vi "Do Action.vi"(7 "Assert Service Enqueuer":refnum<class "Message Enqueuer.lvclass">, 8 "error in (no error)":errorcluster, 11 "UDP Listener in":refnum<class "UDP Listener.lvclass">) -> (0 "error out":errorcluster, 3 "UDP Listener out":refnum<class "UDP Listener.lvclass">)   [LabVIEW 2016, in "Assert API Components.lvlib" / "Assert Service.lvlib" / "UDP Listener.lvclass"]
uses:
  UDP Listener.lvclass
  C:/Users/ukhornp/Documents/Projects/actor_assert_api/Core/Assert Service/Service Actions/Service Action Base.lvclass
  <vilib>/ActorFramework/Message Enqueuer/Message Enqueuer.lvclass
  UDP Listener.lvclass/UDP Listener.ctl
  <vilib>/NI/STM/SubVIs/MetaDataElement.ctl
  Assert Service Messages/New P2P UDP Link Msg/New P2P UDP Link Msg.lvclass/New P2P UDP Link Msg.ctl
  <vilib>/ActorFramework/Message Enqueuer/Message Enqueuer.lvclass/Message Enqueuer.ctl
  <vilib>/NI/STM/UDP/Write Meta Data (UDP Ref).vi
  <vilib>/NI/STM/UDP/Get Connection Reference (UDP).vi
  <vilib>/ActorFramework/Message Enqueuer/Enqueue.vi
  Assert Service Messages/New P2P UDP Link Msg/New P2P UDP Link Msg.lvclass
  C:/Program Files (x86)/National Instruments/LabVIEW 2016/vi.lib/ActorFramework/Message/Message.lvclass
  <vilib>/NI/STM/UDP/Write Meta Data (UDP Clst).vi
  <vilib>/NI/STM/UDP/Read Message (UDP).vi
  <vilib>/NI/STM/UDP/Write Message (UDP).vi
  <vilib>/Utility/LVClass/Get LV Class Name.vi
  <resource>/AFDebug/Generate Trace for Message.vi
  <vilib>/ActorFramework/Message Priority Queue/Priority Enqueue.vi
  <vilib>/NI/STM/NI STM.lvlib
  Service Action Base.lvclass
panel:
  out "data string":string
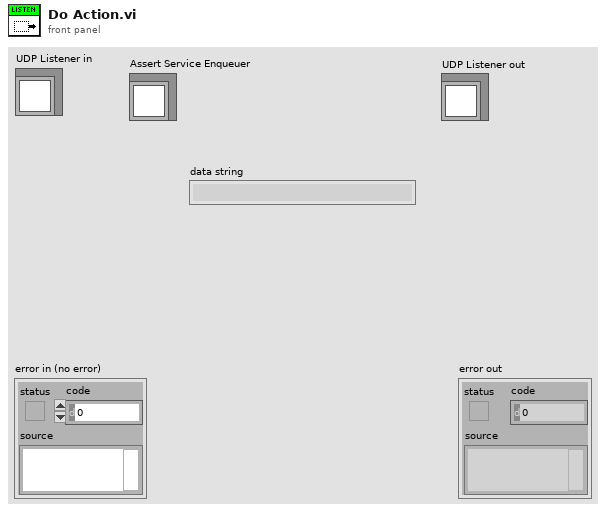
[diagram p1: front panel]
types:
  T1 = typedef "NI STM.lvlib/MetaDataElement.ctl" = string
  T2 = typedef "NI STM.lvlib/UDP Connection Info.ctl" = cluster{"connection ID":refnum<k16>, "meta data":T1[]}
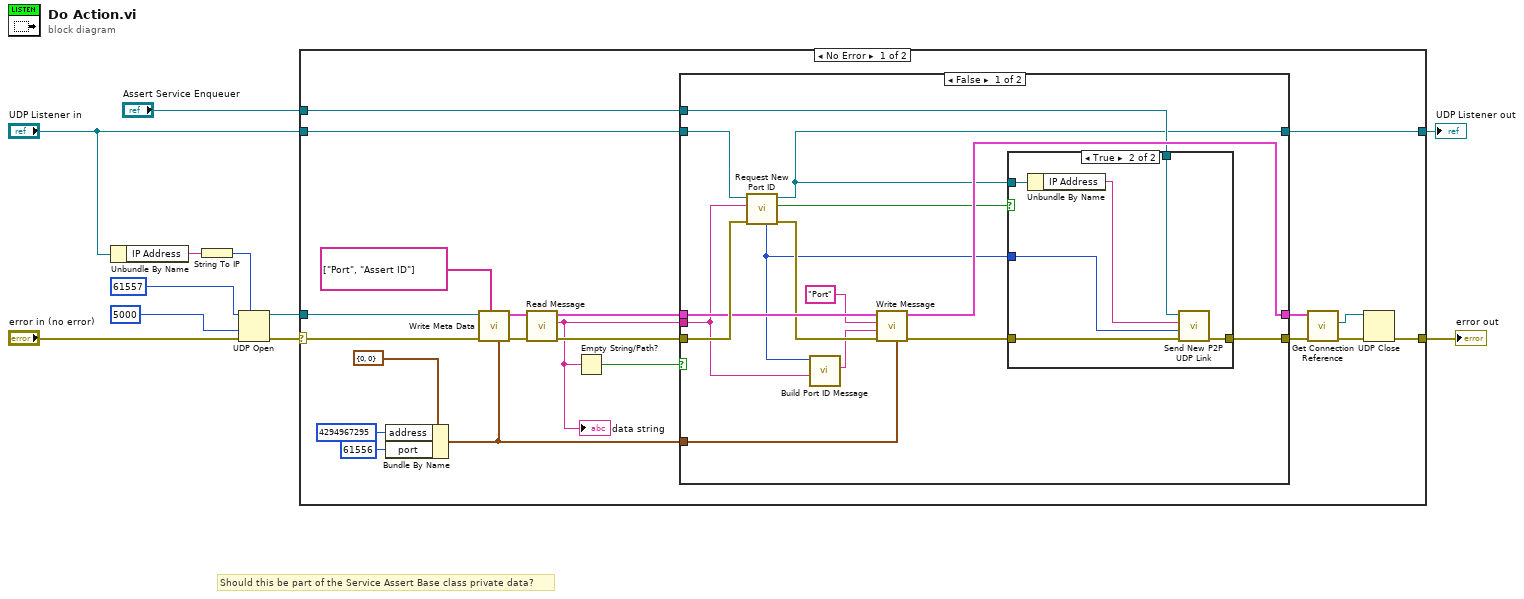
[diagram p0: block diagram]
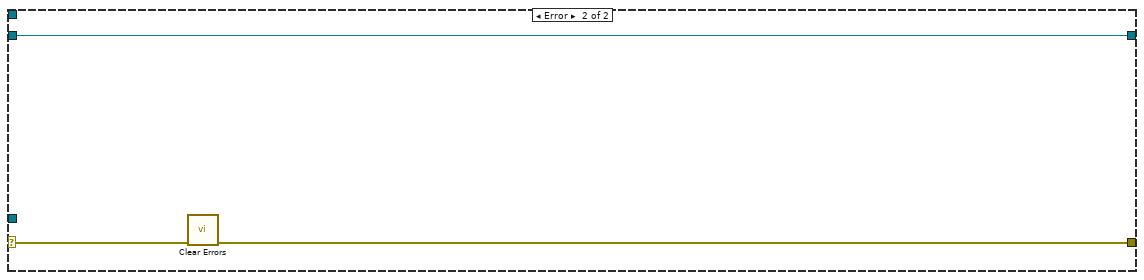
[diagram p4: hidden frame]
diagram:
  # "Should this be part of the Service Assert Base class private data?"
  n1 = Unbundle By Name("UDP Listener in") -> ("IP Address"=w7:string)
  n2 = String To IP(1:w7) -> (0:w11:u32)
  n3 = UDP Open(7:w11, 8:"error in (no error)", 9:5000 ("timeout ms (25000)"), 11:u16 61557 ("port")) -> (port=w5:refnum<k16>, 0:w6:errorcluster)  [unwired: 1 in, 1 out]
  n4 = case shown="No Error" w6 {
    selector: w6 -> [w32 w60]
    tunnel: w5 -> [w31 _]
    tunnel: [w21 w59] -> w4
    tunnel: "UDP Listener in" -> [w14 w58]
    tunnel: [w13 w58] -> w2
    tunnel: "Assert Service Enqueuer" -> [w12 _]
    frame No Error {
      n5 = Bundle By Name(cluster=cluster{"address":u32, "port":u16} {"address"=0, "port"=0} ("address"), "address"=u32 4294967295, "port"=u16 61556) -> (w20:cluster{"address":u32, "port":u16})
      n6 = call-poly <vilib>:"Write Meta Data.vi"("address"=w20, "meta data"=T1[] ["Port", "Assert ID"], "error in"=w32, "connection ID"=w31) -> ("error out"=w22:errorcluster, "connection info out"=w18:T2)  [unwired: 6 in]
      n7 = call-poly <vilib>:"Read Message.vi"("error in"=w22, "connection info in"=w18) -> ("error out"=w19:errorcluster, "data string"=w15:string, "connection info out"=w17:T2)  [unwired: 4 in, 3 out]
      "data string" <- w15
      n8 = Empty String/Path?(string/path=w15) -> (empty?=w16:bool)
      n9 = case shown="False" w16 {
        tunnel: [w47 w55] -> w26
        tunnel: [w37 w56] -> w25
        tunnel: w20 -> [w46 _]
        tunnel: w19 -> [w45 w56]
        tunnel: w17 -> [w44 w55]
        tunnel: w15 -> [w34 _]
        tunnel: w14 -> [w42 w57]
        tunnel: [w36 w57] -> w13
        tunnel: w12 -> [w39 _]
        frame False {
          n10 = call "Request New Port ID.vi"("error in"=w45, "Assert ID"=w34, "Service Action Base in"=w42) -> ("error out"=w43:errorcluster, "Create New Link"=w40:bool, "Service Action Base out"=w36:refnum<class "UDP Listener.lvclass">, "New Port Number"=w33:u16)  [unwired: 5 in]
          n11 = call "Build Port ID Message.vi"("Assert ID String"=w34, "New Port Number"=w33) -> ("Assert Port ID Message"=w35:string)  [unwired: 9 in]
          n12 = call-poly <vilib>:"Write Message.vi"("address"=w46, "error in"=w43, "data"=w35, "name"="Port", "connection info in"=w44) -> ("error out"=w38:errorcluster, "connection info out"=w47:T2)  [unwired: 5 in]
          n13 = case shown="True" w40 {
            tunnel: w39 -> [_ w52]
            tunnel: w38 -> [w48 w54]
            tunnel: [w48 w53] -> w37
            tunnel: w33 -> [_ w51]
            tunnel: w36 -> [_ w50]
            frame False {
            }
            frame True {
              n14 = Unbundle By Name(w50) -> ("IP Address"=w49:string)
              n15 = call "Send New P2P UDP Link.vi"("error in (no error)"=w54, "Port Number"=w51, "IP Address"=w49, "Message Enqueuer"=w52) -> ("error out"=w53:errorcluster)  [unwired: 6 in, 1 out]
            }
          }
        }
        frame True {
        }
      }
      n16 = call-poly <vilib>:"Get Connection Reference.vi"("error in"=w25, "connection info in"=w26) -> ("error out"=w23:errorcluster, "connection ID"=w24:refnum<k16>)  [unwired: 7 in, 1 out]
      n17 = UDP Close(connection ID=w24, 8:w23) -> (error out=w21:errorcluster)  [unwired: 1 out]
    }
    frame Error {
      n18 = call <vilib>:"Clear Errors.vi"("error in (no error)"=w60) -> ("error out"=w59:errorcluster)  [unwired: 5 in, 1 out]
    }
  }
  "error out" <- w4
  "UDP Listener out" <- w2
